vi "HVBuncher.Close.vi"(0 "i ref in":refnum<vi>, 3 "ms timeout (10000)":i32=10000, 5 "error in (no error)":errorcluster) -> (14 "i ref out":refnum<vi>, 17 "timed out":bool, 19 "error out":errorcluster)   [LabVIEW 2014, in "HVBuncher.lvlib"]
doc: "This vi unloads the previously created objects."
uses:
  HVBuncher.lvlib
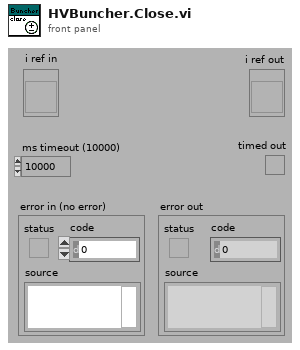
[diagram p1: front panel]
types:
  T1 = typedef "HVBuncher.lvlib/HVBuncher.i attribute.ctl" = cluster{"ObjectsInitialized":bool, "ChildObjects":T2}
  T2 = typedef "HVBuncher.lvlib/HVBuncher.ChildObjects.ctl" = cluster{"ObjectsLoaded":string[], "actVoltage":dbl[]}
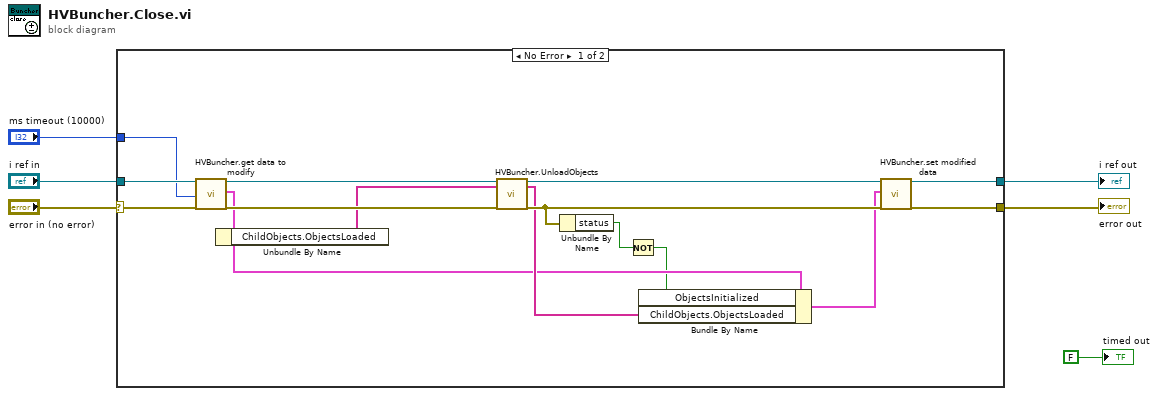
[diagram p0: block diagram]
diagram:
  n1 = case shown="No Error" "error in (no error)" {
    selector: "error in (no error)" -> [w20 w22]
    tunnel: "i ref in" -> [w21 w23]
    tunnel: [w17 w23] -> w5
    tunnel: [w16 w22] -> w3
    tunnel: "ms timeout (10000)" -> [w19 _]
    frame No Error {
      n2 = call "HVBuncher.get data to modify.vi"("i ref in"=w21, "ms timeout (10000)"=w19, "error in (no error)"=w20) -> ("i ref out"=w13:refnum<vi>, "i attribute"=w9:T1, "error out"=w12:errorcluster)  [unwired: 13 in, 1 out]
      n3 = Unbundle By Name(w9) -> ("ChildObjects.ObjectsLoaded"=w11:string[])
      n4 = call "HVBuncher.UnloadObjects.vi"("i ref in"=w13, "ObjectsLoaded in"=w11, "error in (no error)"=w12) -> ("i ref out"=w18:refnum<vi>, "ObjectsLoaded out"=w14:string[], "error out"=w15:errorcluster)  [unwired: 14 in]
      n5 = Unbundle By Name(w15) -> ("status"=w10:bool)
      n6 = Not(x=w10) -> (.not. x?=w7:bool)
      n7 = Bundle By Name(cluster=w9, "ObjectsInitialized"=w7, "ChildObjects.ObjectsLoaded"=w14) -> (w8:T1)
      n8 = call "HVBuncher.set modified data.vi"("i ref in"=w18, "i attribute"=w8, "error in (no error)"=w15) -> ("i ref out"=w17:refnum<vi>, "error out"=w16:errorcluster)  [unwired: 15 in]
    }
    frame Error {
    }
  }
  "error out" <- w3
  "i ref out" <- w5
  "timed out" <- FALSE ("timed out")
